vi "ADQ214 Send Long Processor Command.vi"(5 "data":i32, 6 "mask":i32, 7 "addr":i32, 8 "error in (no error)":errorcluster, 9 "command":i32, 10 "adq214_num":i32, 11 "adq_cu_ptr":u32) -> (0 "error out":errorcluster, 2 "function return":u32, 3 "adq_cu_ptr out":u32)   [LabVIEW 8.6, in "ADQAPI.lvlib"]
doc: "extern \"C\" __declspec(dllimport) unsigned int ADQ214_SendLongProcessorCommand(void* adq_cu_ptr, int adq214_num, int command, int addr, int mask, int data);"
uses:
  F/HRT/Sp Devices Thesis/ADQ-214 project (H R)/ADQAPI.lvlib
  F:/HRT/Sp Devices Thesis/ADQ-214 project (H R)/ADQAPI.dll
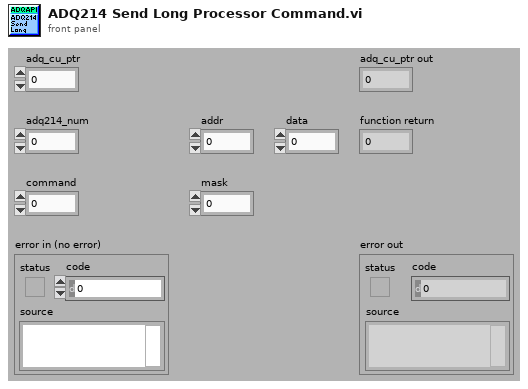
[diagram p1: front panel]
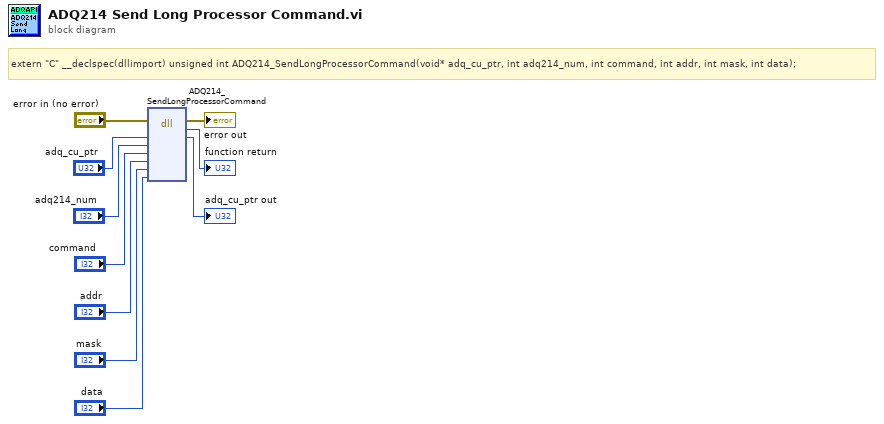
[diagram p0: block diagram]
diagram:
  # "extern \"C\" __declspec(dllimport) unsigned int\tADQ214_SendLongProcessorCommand(void* adq_cu_ptr, int adq214_num, int command, int addr, int mask, int data);"
  n1 = dll-call lib="F:/HRT/Sp Devices Thesis/ADQ-214 project (H R)/ADQAPI.*" fn="ADQ214_SendLongProcessorCommand"(error in="error in (no error)", "adq_cu_ptr"="adq_cu_ptr", "adq214_num"="adq214_num", "command"="command", "addr"="addr", "mask"="mask", "data"="data") -> (error out=→"error out":errorcluster, →"function return":u32, "adq_cu_ptr"=→"adq_cu_ptr out":u32)  [unwired: 7 in, 1 out]
